vi "fitParamExtraction.vi"(6 "startFit":bool, 7 "inputValid":bool, 8 "startIndex":u16, 9 "fittingParams":T4={"maxLoc"=0, "threshold"=0, "fitHardPtLimit"=5000}, 11 "waveLength":u16=5000) -> (0 "minValues":T1, 1 "integralParts":T2, 2 "fitFwd":T3, 3 "fitBwd":T3, 4 "debugOut":cluster{"index":u16, "minimum":i16})   [LabVIEW 2016]
uses:
  <vilib>/rvi/Memory/Memory_Emulation/nirvimemoryFastEmulation.vi
  <vilib>/rvi/Memory/Memory_Emulation/nirvimemoryEmulation.vi
  <vilib>/rvi/Emulation/niFpgaEmulationIsFPGAContextNoSignature.vi
  <vilib>/rvi/DataTransferAndStorage/Container/Common/niFpgaContainerGetUniqueNameForEmu.vi
  <vilib>/rvi/Emulation/niFpgaProcessEmulError.vi
  <vilib>/rvi/Emulation/niFpgaSctlEmulationGetInTimedLoop.vi
  <vilib>/rvi/errors/nirviReportUnexpectedCaseInternalError (U32).vi
  <vilib>/rvi/FXPMathLib/FxpInterpret/XNode/nifxpmath_Interpret.xnode
  <vilib>/rvi/DataTransferAndStorage/Container/XNode/niFpgaContainer.xnode
  <instrlib>/_niInstr/Basic Elements/v1/FPGA/niInstr Basic Elements v1 FPGA.lvlib
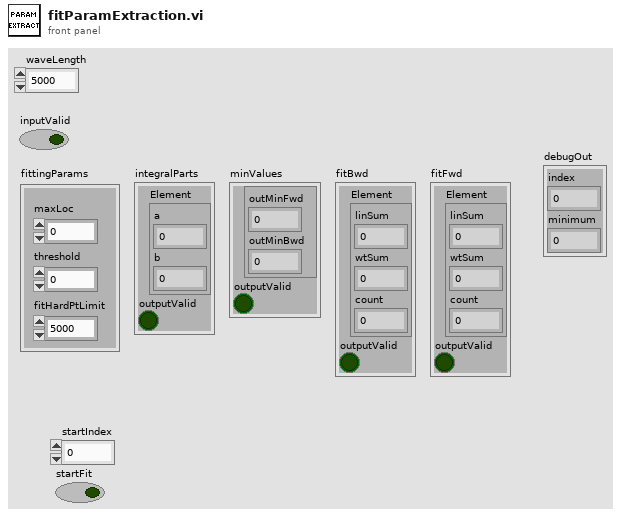
[diagram p1: front panel]
types:
  T1 = cluster{cluster{"outMinFwd":fxp<+/-,22,1>, "outMinBwd":fxp<+/-,22,1>}, "outputValid":bool}
  T2 = cluster{"Element":cluster{"a":i32, "b":i32}, "outputValid":bool}
  T3 = cluster{"Element":cluster{"linSum":i32, "wtSum":fxp<+/-,54,34>, "count":u16}, "outputValid":bool}
  T4 = cluster{"maxLoc":u16, "threshold":i16, "fitHardPtLimit":u16}
  T5 = cluster{"outMinFwd":fxp<+/-,22,1>, "outMinBwd":fxp<+/-,22,1>}
  T6 = cluster{"linSum":i32, "wtSum":fxp<+/-,54,34>, "count":u16}
  T7 = cluster{"Element":cluster{"linSum":i32, "wtSum":fxp<+/-,54,34>, "count":u16}, "edge detected":bool}
  T8 = cluster{"Element":cluster{"a":i32, "b":i32}, bool}
  T9 = cluster{cluster{"outMinFwd":fxp<+/-,22,1>, "outMinBwd":fxp<+/-,22,1>}, bool}
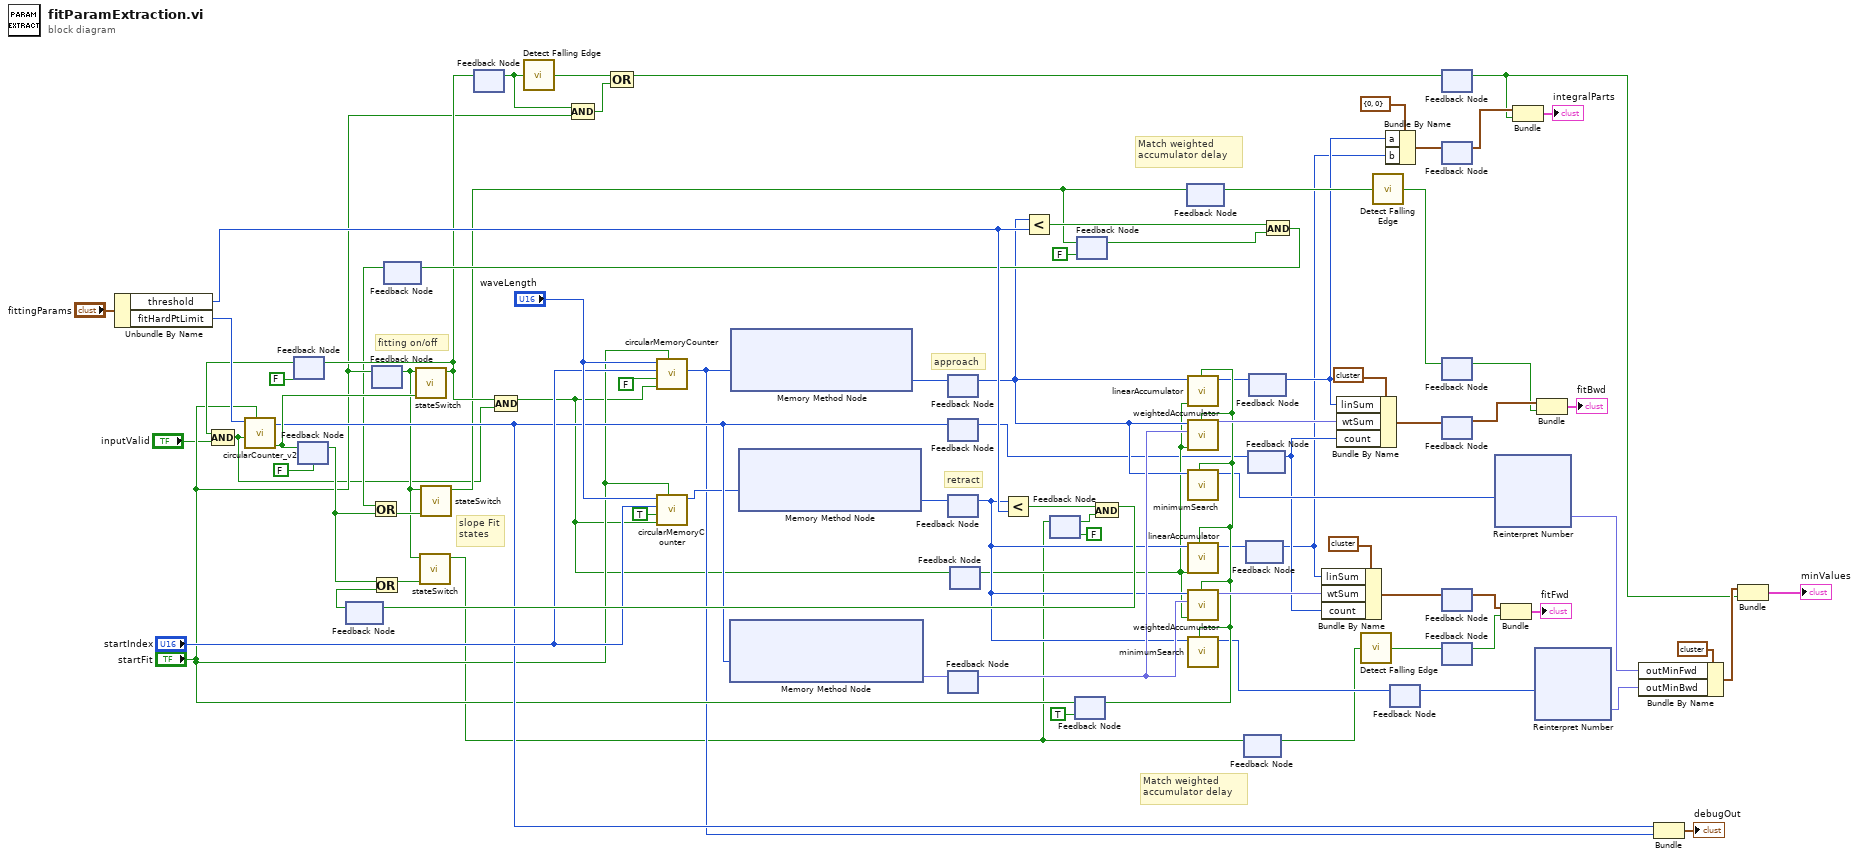
[diagram p0: block diagram]
diagram:
  # "Match weighted accumulator delay"
  # "Match weighted accumulator delay"
  # "fitting on/off"
  # "slope Fit\nstates"
  # "retract"
  # "approach"
  n1 = Unbundle By Name("fittingParams") -> ("threshold"=w76:i16, "fitHardPtLimit"=w83:u16)
  n2 = feedback #1(FALSE) -> (w79:bool)
  n3 = Compound Arithmetic op=AND(w79, "inputValid") -> (w5:bool)
  n4 = call "circularCounter_v2.vi"("reset"="startFit", "doStep"=w5, "maxCount"=w83) -> ("maxReached"=w54:bool, "index"=w27:u16)  [unwired: 5 in, 2 out]
  n5 = feedback #2(FALSE ("maxReached")) -> (w60:bool)
  n6 = feedback-in #2(w54) -> ()
  n7 = feedback #3() -> (w19:bool)  [unwired: 1 in]
  n8 = feedback-in #4("startFit") -> ()
  n9 = feedback #4() -> (w20:bool)  [unwired: 1 in]
  n10 = Or(x=w60, y=w19) -> (x .or. y?=w77:bool)
  n11 = feedback #5() -> (w18:bool)  [unwired: 1 in]
  n12 = Or(x=w18, y=w60) -> (x .or. y?=w78:bool)
  n13 = call "stateSwitch.vi"("disable"=w54, "enable"=w20) -> ("state"=w52:bool)  [unwired: 9 in]
  n14 = feedback-in #1(w52) -> ()
  n15 = call "stateSwitch.vi"("disable"=w77, "enable"=w20) -> ("state"=w11:bool)  [unwired: 9 in]
  n16 = call "stateSwitch.vi"("disable"=w78, "enable"=w20) -> ("state"=w9:bool)  [unwired: 9 in]
  n17 = feedback #6() -> (w23:bool)  [unwired: 1 in]
  n18 = feedback-in #6(w52) -> ()
  n19 = Compound Arithmetic op=AND(w52, w5) -> (w13:bool)
  n20 = call <instrlib>:"Detect Falling Edge.vi"("signal"=w23) -> ("edge detected"=w53:bool)  [unwired: 14 in]
  n21 = Compound Arithmetic op=AND(w23, "startFit") -> (w21:bool)
  n22 = Compound Arithmetic op=OR(w53, w21) -> (w24:bool)
  n23 = call "circularMemoryCounter.vi"("reset"="startFit", "doStep"=w13, "foward"=FALSE, "start"="startIndex", "maxCount"="waveLength") -> ("next"=w15:u16)  [unwired: 4 in, 2 out]
  n24 = call "circularMemoryCounter.vi"("reset"="startFit", "doStep"=w13, "foward"=TRUE, "start"="startIndex", "maxCount"="waveLength") -> ("index"=w16:u16)  [unwired: 4 in, 2 out]
  n25 = xnode ("Memory Method Node")("Address"=w27) -> ("Data"=w81:fxp<+,16,0>)  [unwired: 1 in, 1 out]
  n26 = xnode ("Memory Method Node")("Address"=w15) -> ("Data"=w82:i16)  [unwired: 1 in, 1 out]
  n27 = xnode ("Memory Method Node")("Address"=w16) -> ("Data"=w69:i16)  [unwired: 1 in, 1 out]
  n28 = feedback #7() -> (w47:i16)  [unwired: 1 in]
  n29 = feedback-in #7(w82) -> ()
  n30 = feedback #8() -> (w3:u16)  [unwired: 1 in]
  n31 = feedback-in #8(w27) -> ()
  n32 = feedback #9() -> (w17:i16)  [unwired: 1 in]
  n33 = feedback-in #9(w69) -> ()
  n34 = feedback #10() -> (w80:fxp<+,16,0>)  [unwired: 1 in]
  n35 = feedback-in #10(w81) -> ()
  n36 = feedback #11() -> (w12:bool)  [unwired: 1 in]
  n37 = feedback-in #11(w13) -> ()
  n38 = Less?(x=w17, y=w76) -> (x < y?=w70:bool)
  n39 = Less?(x=w47, y=w76) -> (x < y?=w71:bool)
  n40 = feedback #12(FALSE ("state")) -> (w61:bool)
  n41 = feedback-in #12(w11) -> ()
  n42 = feedback #13(TRUE ("Output Valid")) -> (w55:bool)
  n43 = feedback-in #13("startFit") -> ()
  n44 = feedback #14(FALSE ("state")) -> (w65:bool)
  n45 = feedback-in #14(w9) -> ()
  n46 = And(x=w70, y=w61) -> (x .and. y?=w62:bool)
  n47 = feedback-in #3(w62) -> ()
  n48 = feedback #15() -> (w8:bool)  [unwired: 1 in]
  n49 = feedback-in #15(w9) -> ()
  n50 = call "linearAccumulator.vi"("reset"=w55, "inputValid"=w12, "input"=w47) -> ("sum"=w7:i32)  [unwired: 6 in, 1 out]
  n51 = call "weightedAccumulator.vi"("reset"=w55, "inputValid"=w12, "weight"=w80, "input"=w47) -> ("weightedSum"=w75:fxp<+/-,54,34>)  [unwired: 6 in, 1 out]
  n52 = call "minimumSearch.vi"("reset"=w55, "input"=w47) -> ("minimum"=w34:i16)  [unwired: 9 in]
  n53 = call "linearAccumulator.vi"("reset"=w55, "inputValid"=w12, "input"=w17) -> ("sum"=w4:i32)  [unwired: 6 in, 1 out]
  n54 = call "weightedAccumulator.vi"("reset"=w55, "inputValid"=w12, "weight"=w80, "input"=w17) -> ("weightedSum"=w74:fxp<+/-,54,34>)  [unwired: 6 in, 1 out]
  n55 = call "minimumSearch.vi"("reset"=w55, "input"=w17) -> ("minimum"=w26:i16)  [unwired: 9 in]
  n56 = feedback #16() -> (w10:bool)  [unwired: 1 in]
  n57 = feedback-in #16(w11) -> ()
  n58 = feedback #17() -> (w1:i32)  [unwired: 1 in]
  n59 = feedback-in #17(w4) -> ()
  n60 = feedback #18() -> (w2:u16)  [unwired: 1 in]
  n61 = feedback-in #18(w3) -> ()
  n62 = feedback #19() -> (w6:i32)  [unwired: 1 in]
  n63 = feedback-in #19(w7) -> ()
  n64 = And(x=w71, y=w65) -> (x .and. y?=w66:bool)
  n65 = feedback-in #5(w66) -> ()
  n66 = Bundle By Name(cluster=T6 {"linSum"=0, "wtSum"=0.0, "count"=0} ("Element"), "linSum"=w1, "wtSum"=w74, "count"=w2) -> (w72:T6)
  n67 = Bundle By Name(cluster=T6 {"linSum"=0, "wtSum"=0.0, "count"=0} ("Element"), "linSum"=w6, "wtSum"=w75, "count"=w2) -> (w73:T6)
  n68 = call <instrlib>:"Detect Falling Edge.vi"("signal"=w10) -> ("edge detected"=w68:bool)  [unwired: 14 in]
  n69 = call <instrlib>:"Detect Falling Edge.vi"("signal"=w8) -> ("edge detected"=w67:bool)  [unwired: 14 in]
  n70 = Bundle By Name(cluster=cluster{"a":i32, "b":i32} {"a"=0, "b"=0} ("Element"), "a"=w6, "b"=w1) -> (w50:cluster{"a":i32, "b":i32})
  n71 = feedback #20() -> (w36:i16)  [unwired: 1 in]
  n72 = feedback-in #20(w26) -> ()
  n73 = feedback #21() -> (w31:bool)  [unwired: 1 in]
  n74 = feedback-in #21(w24) -> ()
  n75 = feedback #22() -> (w38:cluster{"a":i32, "b":i32})  [unwired: 1 in]
  n76 = feedback-in #22(w50) -> ()
  n77 = feedback #23() -> (w40:bool)  [unwired: 1 in]
  n78 = feedback-in #23(w67) -> ()
  n79 = feedback #24() -> (w41:T6)  [unwired: 1 in]
  n80 = feedback-in #24(w73) -> ()
  n81 = feedback #25() -> (w45:T6)  [unwired: 1 in]
  n82 = feedback-in #25(w72) -> ()
  n83 = feedback #26() -> (w44:bool)  [unwired: 1 in]
  n84 = feedback-in #26(w68) -> ()
  n85 = xnode "Reinterpret Number"("x"=w34) -> ("y"=w33:fxp<+/-,16,1>)
  n86 = Bundle("Element"=w45, "edge detected"=w44) -> (→"fitFwd":T7)  [unwired: 1 in]
  n87 = Bundle("Element"=w38, w31) -> (→"integralParts":T8)  [unwired: 1 in]
  n88 = xnode "Reinterpret Number"("x"=w36) -> ("y"=w35:fxp<+/-,16,1>)
  n89 = Bundle("Element"=w41, "edge detected"=w40) -> (→"fitBwd":T7)  [unwired: 1 in]
  n90 = Bundle By Name(cluster=T5 {"outMinFwd"=0.0, "outMinBwd"=0.0}, "outMinFwd"=w33, "outMinBwd"=w35) -> (w32:T5)
  n91 = Bundle("index"=w27, "next"=w15) -> (→"debugOut":cluster{"index":u16, "next":u16})  [unwired: 1 in]
  n92 = Bundle(w32, w31) -> (→"minValues":T9)  [unwired: 1 in]
